vi "Main.vi"() -> ()   [LabVIEW 2015, in "Collect Data Mgr.lvlib"]
doc: "This template is based from the Queued Message Handler design pattern and the Queued Message Handler Project Template that ships with LabVIEW 2014.\n\nThe main difference is that the Queue is private to this module and communication between modules is done via Broadcast and Request events.\n\nRequest events are wrapped via public API methods and are handled in the Event handler loop in this VI.\nAny module can register for Broadcast events sent by this module.\n\nThe Event Handling Loop generates messages based on user interface actions.\n\nThe Message Handling Loop processes messages generated by the Event Handling Loop, or by other messages. The messages are string values, so new messages can be added easily to the Message Cases case structure in the Message Handling Loop. Each message cluster can also provide an optional value for Message Data, which is a variant that can be converted to whatever message-specific data is required.\n_____\nBased on Delacor QMH Project Template 2.1.0.2."
uses:
  Collect Data Mgr.lvlib
  <vilib>/Delacor/Delacor QMH/Libraries/Module Admin_class/Delacor_lib_QMH_Module Admin.lvclass
  Module Data--cluster.ctl
  <vilib>/Delacor/Delacor QMH/Libraries/Message Queue_class/Delacor_lib_QMH_Message Queue.lvclass/Delacor_lib_QMH_Message Queue.ctl
  Stop Argument--cluster.ctl
  <vilib>/Delacor/Delacor QMH/Libraries/Module Admin_class/Delacor_lib_QMH_Module Admin.lvclass/Delacor_lib_QMH_Module Admin.ctl
  Start Collect Argument--cluster.ctl
  Start Collect (Reply Payload)--cluster.ctl
  Stop Collect Argument--cluster.ctl
  Stop Collect (Reply Payload)--cluster.ctl
  Tool Interface/_HS Data Stream Params Cluster--typedef.ctl
  <vilib>/Delacor/Delacor QMH/Libraries/Message Queue_class/Delacor_lib_QMH_Enqueue Message (Single).vi
  <vilib>/Delacor/Delacor QMH/Libraries/Module Admin_class/Delacor_lib_QMH_Get External Launch.vi
  <vilib>/Utility/error.llb/Error Cluster From Error Code.vi
  <vilib>/ErrorRing/Error Ring.xnode
  <vilib>/Delacor/Delacor QMH/Libraries/Message Queue_class/Delacor_lib_QMH_Message Queue.lvclass
  Tool Interface/Tool Interface.lvlib
panel:
  in  "Stop":bool
  in  "Simulate MHL Error":bool
  in  "Simulate EHL Error":bool
  out "error out":errorcluster
  in  "Module Admin":refnum<class "Delacor_lib_QMH_Module Admin.lvclass">
  out "Status":string
  # "Other QMH Modules communicate with this Module via its Public API (wrappers for its Request Events).\n\nThis Module communicates with other Modules via its Broadcast Events.\nAny module that wants to get these messages, just registers for this module's Broadcast events."
  # "This template is for the Delacor Modified Queued Message Handler design pattern.\n\nSee the block diagram for more information on how to use this template."
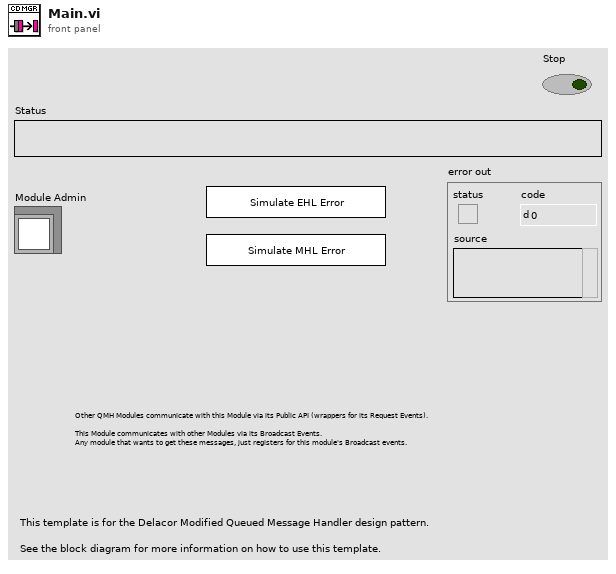
[diagram p1: front panel]
types:
  T1 = typedef "Collect Data Mgr.lvlib/Request Events--cluster.ctl" = cluster{"Stop Module":refnum<user-event>, "Show Panel":refnum<user-event>, "Hide Panel":refnum<user-event>, "Get Module Execution Status":refnum<user-event>, "Show Diagram":refnum<user-event>, "Start Collect":refnum<user-event>, "Stop Collect":refnum<user-event>}
  T2 = typedef "Collect Data Mgr.lvlib/Module Data--cluster.ctl" = cluster{"Status":string, "Error Code":u8, "Data Array DVR":refnum<data-value>, "Sample Data notifier":refnum<notifier>, "Block Count Notifier":refnum<notifier>, "Data Array":u32[][]}
  T3 = typedef "Collect Data Mgr.lvlib/Stop Argument--cluster.ctl" = cluster{"Origin":string, "Exit via Stop Module Req?":bool, "Wait for Module to stop?":bool}
  T4 = typedef "Collect Data Mgr.lvlib/Start Collect Argument--cluster.ctl" = cluster{"Lasers ON?":bool, "Move Length":i32, "Sample Data notifier":refnum<notifier>, "data value reference":refnum<data-value>, "Wait Notifier":refnum<notifier>}
  T5 = typedef "Collect Data Mgr.lvlib/Stop Collect Argument--cluster.ctl" = cluster{"dummy":bool, "Wait Notifier":refnum<notifier>}
  T6 = enum32{"Invalid", "Standard", "Closed", "Hidden", "Minimized", "Maximized"}
  T7 = enum16{"Idle", "Receive HS Data", "Close Connection"}
  T8 = typedef "Tool Interface.lvlib/_HS Data Stream Params Cluster--typedef.ctl" = cluster{"Raw Data Stream Loop cmd":enum16{"Idle", "Receive HS Data", "Close Connection"}, "Data Array DVR ref":refnum<data-value>, "Sample Data notifier":refnum<notifier>, "Block Count Notifier":refnum<notifier>}
  T9 = typedef "Collect Data Mgr.lvlib/Stop Collect (Reply Payload)--cluster.ctl" = cluster{"Success":bool, "CD_Status":i32, "Array Size":u32, "data value reference":refnum<data-value>}
  T10 = typedef "Tool Interface.lvlib/_Loop Ctrl Notifiers Cluster--typedef.ctl" = cluster{"Raw Stream Ctrl":refnum<notifier>}
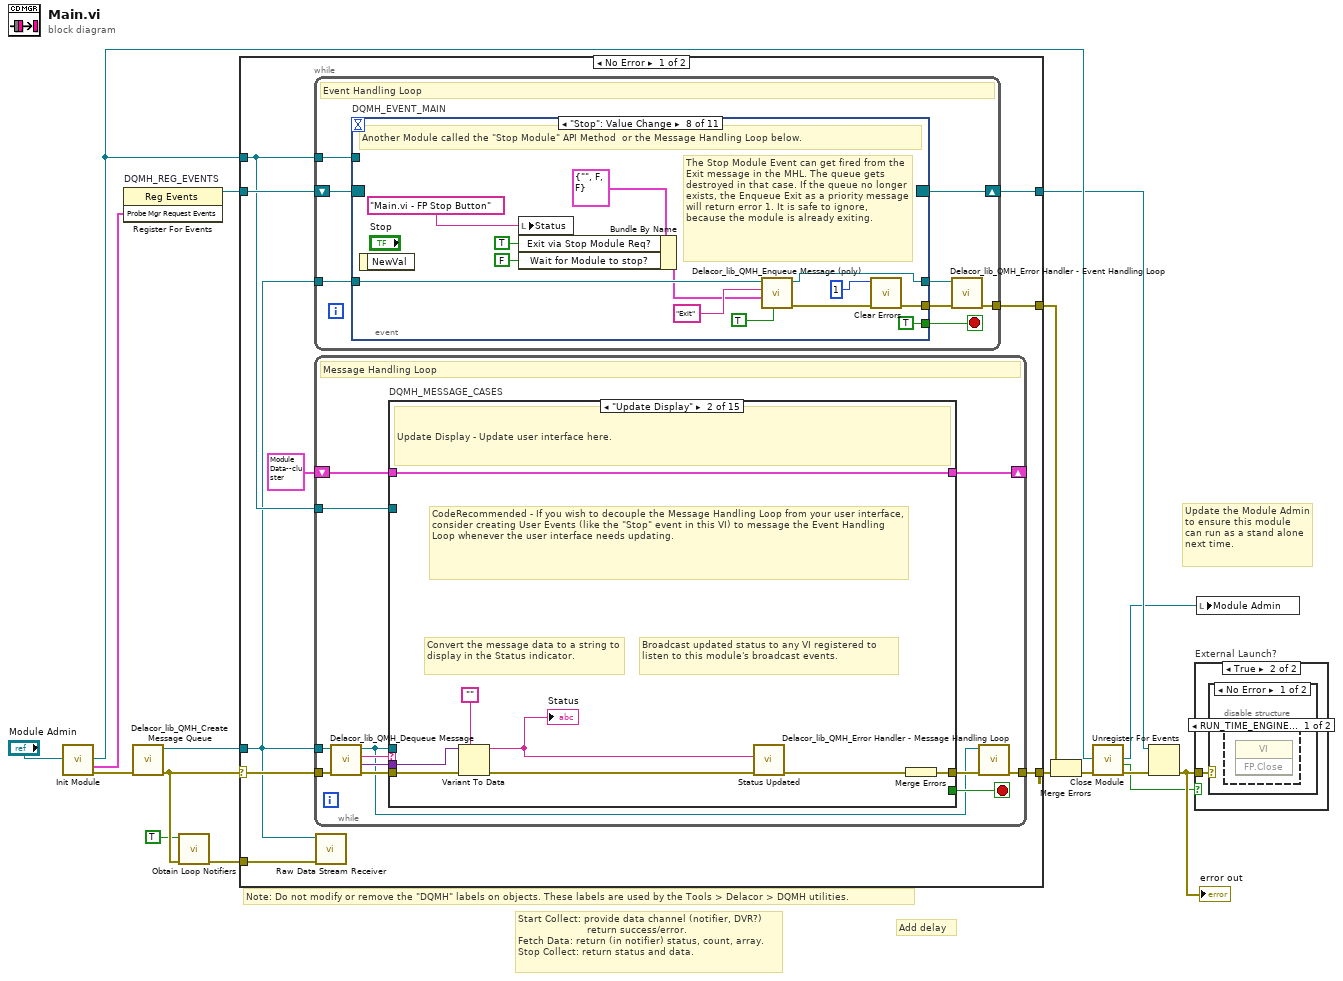
[diagram p0: block diagram]
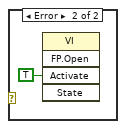
[diagram p4: hidden frame]
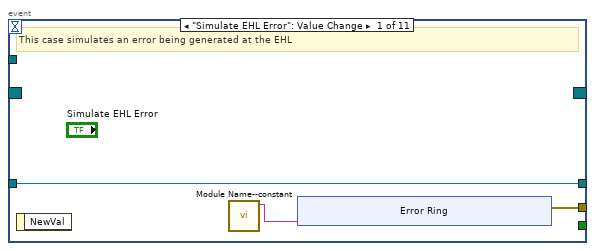
[diagram p5: hidden frame]
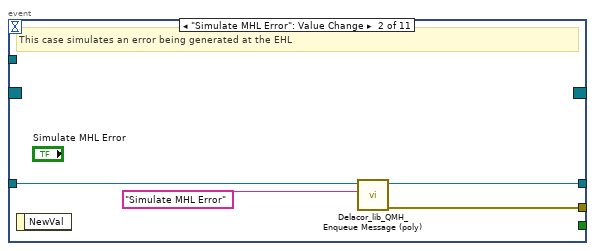
[diagram p6: hidden frame]
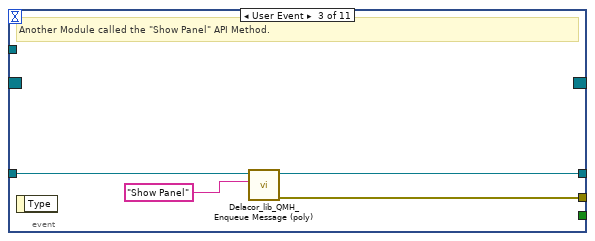
[diagram p7: hidden frame]
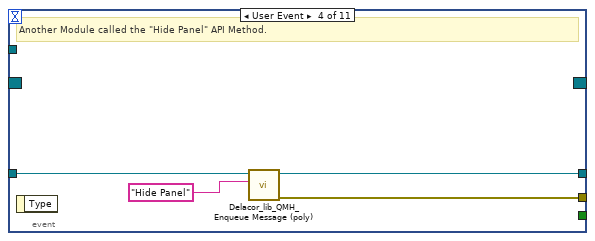
[diagram p8: hidden frame]
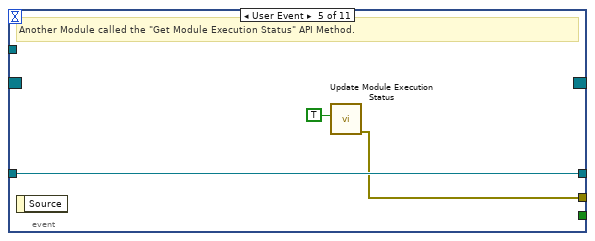
[diagram p9: hidden frame]
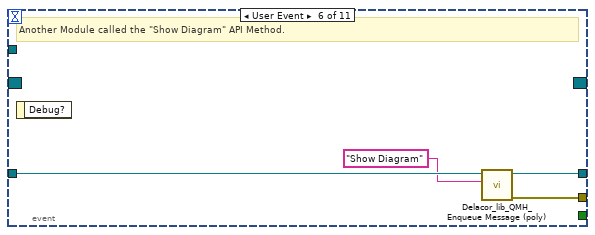
[diagram p10: hidden frame]
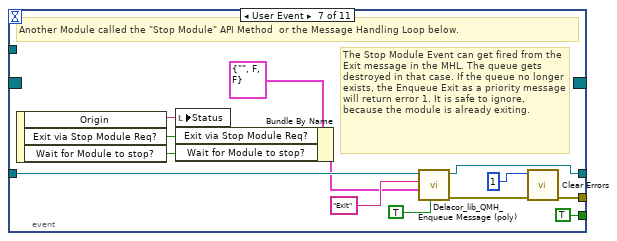
[diagram p11: hidden frame]
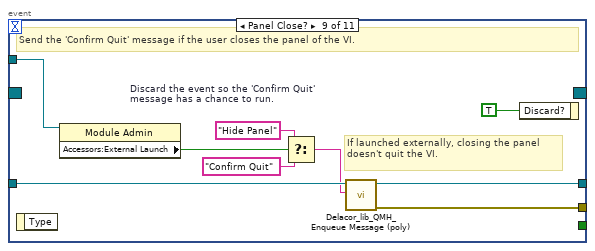
[diagram p12: hidden frame]
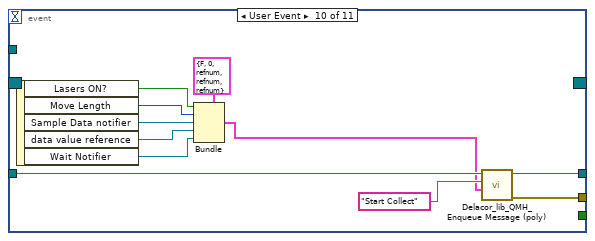
[diagram p13: hidden frame]
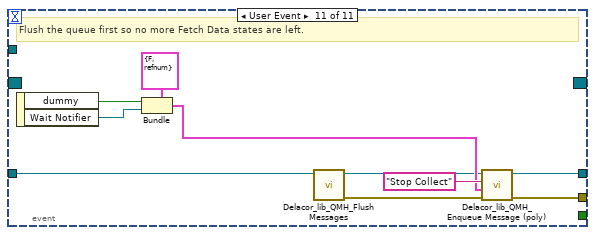
[diagram p14: hidden frame]
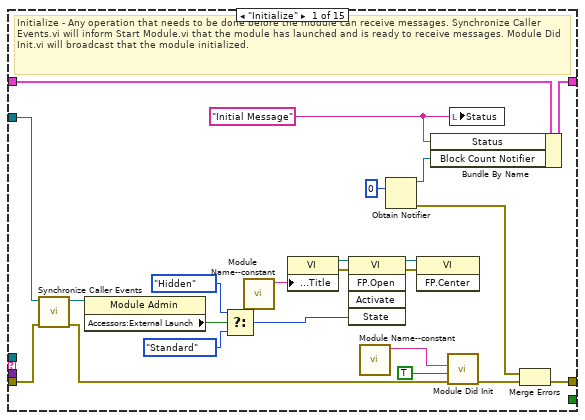
[diagram p15: hidden frame]
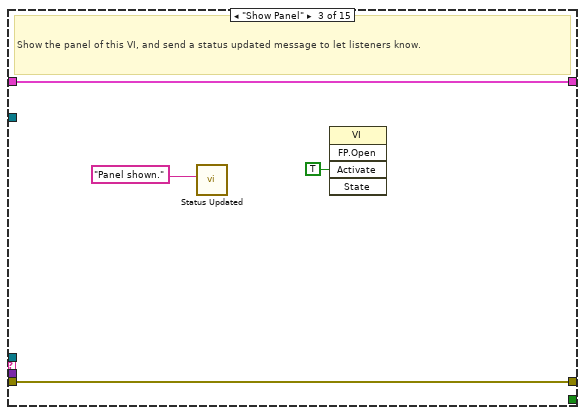
[diagram p16: hidden frame]
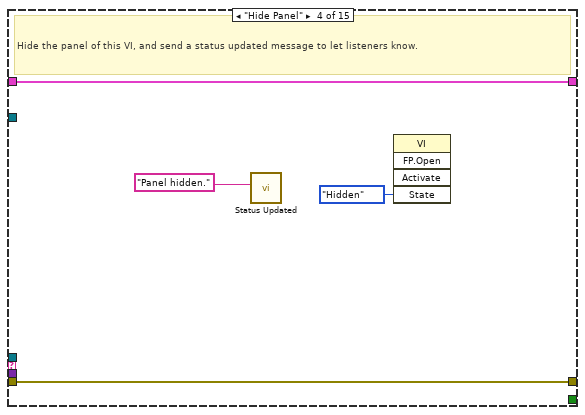
[diagram p17: hidden frame]
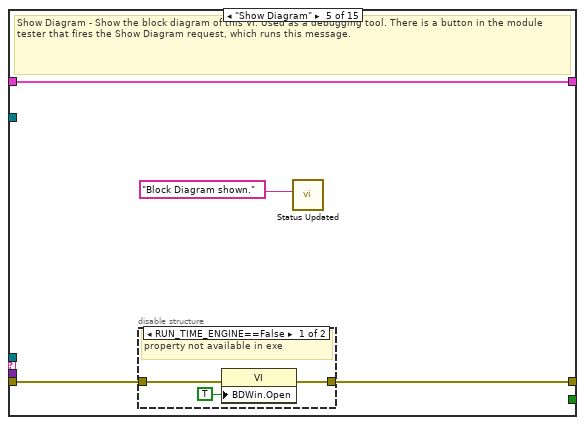
[diagram p18: hidden frame]
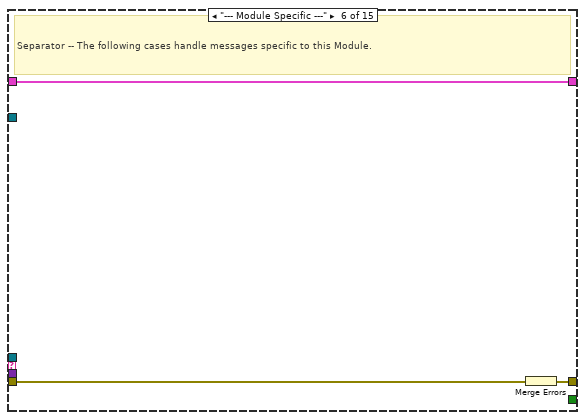
[diagram p20: hidden frame]
diagram:
  # "Add delay"
  # "Start Collect: provide data channel (notifier, DVR?)\n                       return success/error.\nFetch Data: return (in notifier) status, count, array.\nStop Collect: return status and data."
  # "Note: Do not modify or remove the \"DQMH\" labels on objects. These labels are used by the Tools > Delacor > DQMH utilities."
  # "Update the Module Admin to ensure this module can run as a stand alone next time."
  n1 = call "Init Module.vi"("Singleton Module Admin in"="Module Admin") -> ("error out"=w4:errorcluster, "Probe Mgr Request Events"=w13:T1, "Singleton Module Admin out"=w17:refnum<class "Delacor_lib_QMH_Module Admin.lvclass">)  [unwired: 8 in]
  n2 = register-events "DQMH_REG_EVENTS"(w13) -> (reference out=w14:refnum<event-registration>)  [unwired: 2 in, 1 out]
  n3 = call <vilib>:"Delacor_lib_QMH_Create Message Queue.vi"("error in (no error)"=w4) -> ("error out"=w3:errorcluster, "Message Queue"=w12:refnum<class "Delacor_lib_QMH_Message Queue.lvclass">)  [unwired: 9 in]
  n4 = call "Obtain Loop Notifiers.vi"("error in (no error)"=w3, "Create New"=TRUE) -> ("error out"=w1:errorcluster)  [unwired: 8 in, 1 out]
  n5 = case shown="No Error" w3 {
    selector: w3 -> [w21 w310]
    tunnel: [w26 w310] -> w16
    tunnel: [w25 w315] -> w15
    tunnel: w14 -> [w23 w315]
    tunnel: w12 -> [w18 _]
    tunnel: [w22 _] -> w8
    tunnel: w17 -> [w20 w311]
    tunnel: w1 -> [w19 _]
    frame No Error {
      n6 = while {
        tunnel: w18 -> [w34]
        shift-right: [w32] -> w25
        shift-left: w23 -> [w33]
        tunnel: [w28] -> w22
        tunnel: w20 -> [w27]
        stop <- w30 stop-if-true
        # "Event Handling Loop"
        n7 = event "DQMH_EVENT_MAIN" shown="[7] \"Stop\": Value Change" {
          selector: w33 -> [_ _ _ _ _ _ _ _ _ _ _]
          dyn-events: [_ _ _ _ _ _ _ _ _ _ _] -> w32
          timeout: _ -> [_ _ _ _ _ _ _ _ _ _ _]
          tunnel: [_ _ _ _ _ _ TRUE ("Discard?") TRUE ("Discard?") _ _ _] -> w30
          tunnel: w34 -> [w37 w48 w52 w56 w59 w63 w74 w87 w97 w109 w112]
          tunnel: [w36 w45 w50 w54 w58 w60 w68 w82 w96 w104 w115] -> w31
          tunnel: [w37 w47 w51 w55 w59 w62 w73 w86 w95 w108 w119] -> w29
          tunnel: w27 -> [_ _ _ _ _ _ _ _ w91 _ _]
          event "Simulate EHL Error": Value Change {
            # "This case simulates an error being generated at the EHL"
            n8 = event-data() -> ()  [unwired: 1 in, 1 out]
            n9 = call "Module Name--constant.vi"() -> ("Module Name"=w35:string)  [unwired: 11 in]
            n10 = xnode "Error Ring"("parameter 0"=w35) -> ("error out"=w36:errorcluster)
          }
          event "Simulate MHL Error": Value Change {
            # "This case simulates an error being generated at the EHL"
            n11 = event-data() -> ()  [unwired: 1 in, 1 out]
            n12 = call-poly <vilib>:"Delacor_lib_QMH_Enqueue Message (poly).vi"("Message"="Simulate MHL Error", "Message Queue in"=w48) -> ("error out"=w45:errorcluster, "Message Queue out"=w47:refnum<class "Delacor_lib_QMH_Message Queue.lvclass">)  [unwired: 8 in]
          }
          event User Event {
            # "Another Module called the \"Show Panel\" API Method."
            n13 = event-data() -> ()  [unwired: 1 in, 1 out]
            n14 = call-poly <vilib>:"Delacor_lib_QMH_Enqueue Message (poly).vi"("Message"="Show Panel", "Message Queue in"=w52) -> ("error out"=w50:errorcluster, "Message Queue out"=w51:refnum<class "Delacor_lib_QMH_Message Queue.lvclass">)  [unwired: 8 in]
          }
          event User Event {
            # "Another Module called the \"Hide Panel\" API Method."
            n15 = event-data() -> ()  [unwired: 1 in, 1 out]
            n16 = call-poly <vilib>:"Delacor_lib_QMH_Enqueue Message (poly).vi"("Message"="Hide Panel", "Message Queue in"=w56) -> ("error out"=w54:errorcluster, "Message Queue out"=w55:refnum<class "Delacor_lib_QMH_Message Queue.lvclass">)  [unwired: 8 in]
          }
          event User Event {
            # "Another Module called the \"Get Module Execution Status\" API Method."
            n17 = event-data() -> ()  [unwired: 1 in, 1 out]
            n18 = call "Update Module Execution Status.vi"("Running?"=TRUE) -> ("error out"=w58:errorcluster)  [unwired: 10 in]
          }
          event User Event {
            # "Another Module called the \"Show Diagram\" API Method."
            n19 = event-data() -> ()  [unwired: 1 in, 1 out]
            n20 = call-poly <vilib>:"Delacor_lib_QMH_Enqueue Message (poly).vi"("Message"="Show Diagram", "Message Queue in"=w63) -> ("error out"=w60:errorcluster, "Message Queue out"=w62:refnum<class "Delacor_lib_QMH_Message Queue.lvclass">)  [unwired: 8 in]
          }
          event User Event {
            # "The Stop Module Event can get fired from the Exit message in the MHL. The queue gets destroyed in that case. If the queue no longer exists, the Enqueue Exit as a priority message will return error 1. It is safe to ignore, because the module is already exiting."
            # "Another Module called the \"Stop Module\" API Method  or the Message Handling Loop below."
            n21 = event-data() -> ("Origin"=w72:string, "Exit via Stop Module Req?"=w66:bool, "Wait for Module to stop?"=w65:bool)  [unwired: 1 in]
            n22 = local write "Status"(w72) -> ()
            n23 = Bundle By Name(cluster=T3 {"Origin"="", "Exit via Stop Module Req?"=FALSE, "Wait for Module to stop?"=FALSE} ("Stop Argument"), "Exit via Stop Module Req?"=w66, "Wait for Module to stop?"=w65) -> (w64:T3)
            n24 = call-poly <vilib>:"Delacor_lib_QMH_Enqueue Message (poly).vi"("Priority Message? (F)"=TRUE, "Message Data"=w64, "Message"="Exit", "Message Queue in"=w74) -> ("error out"=w69:errorcluster, "Message Queue out"=w73:refnum<class "Delacor_lib_QMH_Message Queue.lvclass">)  [unwired: 6 in]
            n25 = call <vilib>:"Clear Errors.vi"("error in (no error)"=w69, "specific error code to clear (0: all)"=1) -> ("error out"=w68:errorcluster)  [unwired: 4 in, 1 out]
          }
          event "Stop": Value Change {
            # "The Stop Module Event can get fired from the Exit message in the MHL. The queue gets destroyed in that case. If the queue no longer exists, the Enqueue Exit as a priority message will return error 1. It is safe to ignore, because the module is already exiting."
            # "Another Module called the \"Stop Module\" API Method  or the Message Handling Loop below."
            n26 = event-data() -> ()  [unwired: 1 in, 1 out]
            n27 = local write "Status"("Main.vi - FP Stop Button") -> ()
            n28 = Bundle By Name(cluster=T3 {"Origin"="", "Exit via Stop Module Req?"=FALSE, "Wait for Module to stop?"=FALSE} ("Stop Argument"), "Exit via Stop Module Req?"=TRUE, "Wait for Module to stop?"=FALSE) -> (w80:T3)
            n29 = call-poly <vilib>:"Delacor_lib_QMH_Enqueue Message (poly).vi"("Priority Message? (F)"=TRUE, "Message Data"=w80, "Message"="Exit", "Message Queue in"=w87) -> ("error out"=w83:errorcluster, "Message Queue out"=w86:refnum<class "Delacor_lib_QMH_Message Queue.lvclass">)  [unwired: 6 in]
            n30 = call <vilib>:"Clear Errors.vi"("error in (no error)"=w83, "specific error code to clear (0: all)"=1) -> ("error out"=w82:errorcluster)  [unwired: 4 in, 1 out]
          }
          event Panel Close? {
            w98 = TRUE  # Discard the event so the 'Confirm Quit' message has a chance to run.
            # "If launched externally, closing the panel doesn't quit the VI."
            # "Send the 'Confirm Quit' message if the user closes the panel of the VI."
            n31 = event-data() -> ()  [unwired: 1 in, 1 out]
            n32 = property class="Module Admin"(reference=w91) -> ("Accessors:External Launch"=w90:bool)  [unwired: 1 in, 2 out]
            n33 = Select(t="Hide Panel" ("Message"), s=w90, f="Confirm Quit" ("Message")) -> (s? t:f=w92:string)
            n34 = call-poly <vilib>:"Delacor_lib_QMH_Enqueue Message (poly).vi"("Message"=w92, "Message Queue in"=w97) -> ("error out"=w96:errorcluster, "Message Queue out"=w95:refnum<class "Delacor_lib_QMH_Message Queue.lvclass">)  [unwired: 8 in]
            n35 = event-data("Discard?"=w98) -> ()  [unwired: 1 in, 1 out]
          }
          event User Event {
            n36 = event-data() -> ("Lasers ON?"=w103:bool, "Move Length"=w102:i32, "Sample Data notifier"=w101:refnum<notifier>, "data value reference"=w100:refnum<data-value>, "Wait Notifier"=w99:refnum<notifier>)  [unwired: 1 in]
            n37 = Bundle(cluster=T4 {"Lasers ON?"=FALSE, "Move Length"=0, "Sample Data notifier"=refnum, "data value reference"=refnum, "Wait Notifier"=refnum} ("Start Collect Argument"), "Lasers ON?"=w103, "Move Length"=w102, "Sample Data notifier"=w101, "data value reference"=w100, "Wait Notifier"=w99) -> (w105:T4)
            n38 = call-poly <vilib>:"Delacor_lib_QMH_Enqueue Message (poly).vi"("Message Data"=w105, "Message"="Start Collect", "Message Queue in"=w109) -> ("error out"=w104:errorcluster, "Message Queue out"=w108:refnum<class "Delacor_lib_QMH_Message Queue.lvclass">)  [unwired: 7 in]
          }
          event User Event {
            # "Flush the queue first so no more Fetch Data states are left."
            n39 = event-data() -> ("dummy"=w114:bool, "Wait Notifier"=w113:refnum<notifier>)  [unwired: 1 in]
            n40 = Bundle(cluster=T5 {"dummy"=FALSE, "Wait Notifier"=refnum} ("Stop Collect Argument"), "dummy"=w114, "Wait Notifier"=w113) -> (w116:T5)
            n41 = call-dynamic "Delacor_lib_QMH_Flush Messages.vi"("Message Queue in"=w112) -> ("error out"=w110:errorcluster, "Message Queue out"=w111:refnum<class "Delacor_lib_QMH_Message Queue.lvclass">)  [unwired: 7 in, 2 out]
            n42 = call-poly <vilib>:"Delacor_lib_QMH_Enqueue Message (poly).vi"("error in (no error)"=w110, "Message Data"=w116, "Message"="Stop Collect", "Message Queue in"=w111) -> ("error out"=w115:errorcluster, "Message Queue out"=w119:refnum<class "Delacor_lib_QMH_Message Queue.lvclass">)  [unwired: 6 in]
          }
        }
        n43 = call-dynamic "Delacor_lib_QMH_Error Handler - Event Handling Loop.vi"("error in (no error)"=w31, "Message Queue in"=w29) -> ("dup error in"=w28:errorcluster)  [unwired: 8 in, 1 out]
      }
      n44 = while {
        tunnel: w18 -> [w123]
        shift-right: [w129] -> _
        shift-left: T2 {"Status"="", "Error Code"=0, "Data Array DVR"=refnum, "Sample Data notifier"=refnum, "Block Count Notifier"=refnum, "Data Array"=[]} ("Data Cluster") -> [w130]
        tunnel: w21 -> [w127]
        tunnel: [w121] -> w26
        tunnel: w20 -> [w120]
        stop <- w128 stop-if-true
        # "Message Handling Loop"
        n45 = call-dynamic "Delacor_lib_QMH_Dequeue Message.vi"("error in (no error)"=w127, "Message Queue in"=w123) -> ("error out"=w126:errorcluster, "Message Data"=w124:variant, "Message"=w125:string, "Message Queue out"=w122:refnum<class "Delacor_lib_QMH_Message Queue.lvclass">)  [unwired: 6 in]
        n46 = case "DQMH_MESSAGE_CASES" shown="\"Update Display\"" w125 {
          selector: w125 -> [_ _ _ _ _ _ _ _ _ _ _ _ _ _ w297]
          tunnel: w122 -> [_ _ _ _ _ _ _ _ _ _ _ w255 w270 w293 _]
          tunnel: w126 -> [w144 w160 w166 w170 w173 w181 w201 _ w236 w239 w244 w261 w274 w295 _]
          tunnel: [w135 w161 w166 w170 w172 w179 w199 w232 w234 w237 w242 w252 w272 w290 w298] -> w131
          tunnel: w130 -> [w143 w162 w165 w169 w174 w180 w184 w217 w235 w238 w243 w260 w273 w277 w299]
          tunnel: [w142 w162 w165 w169 w174 w180 w183 w217 w235 w238 w243 w260 w273 w277 w299] -> w129
          tunnel: [_ _ _ _ _ _ _ _ _ _ _ _ _ w292 _] -> w128
          tunnel: w124 -> [_ w159 _ _ _ _ w200 w231 _ _ _ w259 _ w289 _]
          tunnel: w120 -> [w145 _ _ _ _ _ _ _ _ _ _ w254 _ w283 _]
          frame "Initialize" {
            w141 = "Initial Message" ("Initial Message")
            # "Initialize - Any operation that needs to be done before the module can receive messages. Synchronize Caller Events.vi will inform Start Module.vi that the module has launched and is ready to receive messages. Module Did Init.vi will broadcast that the module initialized."
            n47 = call "Synchronize Caller Events.vi"("error in (no error)"=w144, "Singleton Module Admin in"=w145) -> ("error out"=w138:errorcluster, "Singleton Module Admin out"=w136:refnum<class "Delacor_lib_QMH_Module Admin.lvclass">)  [unwired: 8 in]
            n48 = property class="Module Admin"(reference=w136) -> ("Accessors:External Launch"=w149:bool)  [unwired: 1 in, 2 out]
            n49 = Select(t=T6."Hidden" ("State"), s=w149, f=T6."Standard" ("State")) -> (s? t:f=w146:T6)
            n50 = call "Module Name--constant.vi"() -> ("Module Name"=w154:string)  [unwired: 11 in]
            n51 = property class="VI"("Front Panel.Title"=w154) -> (reference out=w152:refnum<vi>, error out=w153:errorcluster)  [unwired: 2 in]
            n52 = invoke class="VI" method="FP.Open"(reference=w152, error in=w153, "State"=w146) -> (reference out=w151:refnum<vi>, error out=w150:errorcluster)  [unwired: 2 in, 3 out]
            n53 = call "Module Name--constant.vi"() -> ("Module Name"=w139:string)  [unwired: 11 in]
            n54 = Obtain Notifier(notification data type=u32 0) -> (notifier out=w132:refnum<notifier>, error out=w134:errorcluster)  [unwired: 3 in, 1 out]
            n55 = invoke class="VI" method="FP.Center"(reference=w151, error in=w150) -> ()  [unwired: 1 in, 3 out]
            n56 = Bundle By Name(cluster=w143, "Status"=w141, "Block Count Notifier"=w132) -> (w142:T2)
            n57 = call "Module Did Init.vi"("error in (no error)"=w138, "Initialized?"=TRUE, "Origin"=w139) -> ("error out"=w137:errorcluster)  [unwired: 8 in]
            n58 = local write "Status"(w141) -> ()
            n59 = Merge Errors(w134, w137) -> (w135:errorcluster)
          }
          frame "Update Display" {
            # "Broadcast updated status to any VI registered to listen to this module's broadcast events."
            # "Convert the message data to a string to display in the Status indicator."
            # "CodeRecommended - If you wish to decouple the Message Handling Loop from your user interface, consider creating User Events (like the \"Stop\" event in this VI) to message the Event Handling Loop whenever the user interface needs updating."
            # "Update Display - Update user interface here."
            n60 = Variant To Data(error in=w160, type="", Variant=w159) -> (data=w157:string, error out=w156:errorcluster)
            "Status" <- w157
            n61 = call "Status Updated.vi"("error in (no error)"=w156, "Status"=w157) -> ("error out"=w155:errorcluster)  [unwired: 9 in]
            n62 = Merge Errors(w155) -> (w161:errorcluster)
          }
          frame "Show Panel" {
            # "Show the panel of this VI, and send a status updated message to let listeners know."
            n63 = call "Status Updated.vi"("Status"="Panel shown." ("format string")) -> ()  [unwired: 10 in, 1 out]
            n64 = invoke class="VI" method="FP.Open"("Activate"=TRUE ("Activate?")) -> ()  [unwired: 4 in, 5 out]
          }
          frame "Hide Panel" {
            # "Hide the panel of this VI, and send a status updated message to let listeners know."
            n65 = call "Status Updated.vi"("Status"="Panel hidden." ("format string")) -> ()  [unwired: 10 in, 1 out]
            n66 = invoke class="VI" method="FP.Open"("State"=T6."Hidden") -> ()  [unwired: 4 in, 5 out]
          }
          frame "Show Diagram" {
            # "Show Diagram - Show the block diagram of this VI. Used as a debugging tool. There is a button in the module tester that fires the Show Diagram request, which runs this message."
            n67 = disable-structure shown="RUN_TIME_ENGINE==False" {
              disable-tunnel: [w176 w178] -> w172
              disable-tunnel: w173 -> [w175 w178]
              frame condition #0 (active) {
                # "property not available in exe"
                n68 = property class="VI"(error in=w175, "BDWin.Open"=TRUE ("Block Diagram Window:Open")) -> (error out=w176:errorcluster)  [unwired: 1 in, 1 out]
              }
              frame condition #1 {
              }
            }
            n69 = call "Status Updated.vi"("Status"="Block Diagram shown." ("format string")) -> ()  [unwired: 10 in, 1 out]
          }
          frame "--- Module Specific ---" {
            # "Separator -- The following cases handle messages specific to this Module."
            n70 = Merge Errors(w181) -> (w179:errorcluster)
          }
          frame "Start Collect" {
            # "Set the Mode, move length, and the expected return data array length, and then start the data collection. Save the current VISA timeout value and set it to 1000mSec for data collection. Save the VISA resource name and the DVR ref that holds the full data storage array (passed in from caller)."
            n71 = Variant To Data(error in=w201, type=T4 {"Lasers ON?"=FALSE, "Move Length"=0, "Sample Data notifier"=refnum, "data value reference"=refnum, "Wait Notifier"=refnum} ("Start Collect Argument"), Variant=w200) -> (data=w189:T4, error out=w197:errorcluster)
            n72 = Unbundle By Name(w184) -> ("Block Count Notifier"=w202:refnum<notifier>)
            n73 = Unbundle By Name(w189) -> ("Sample Data notifier"=w192:refnum<notifier>, "data value reference"=w185:refnum<data-value>, "Lasers ON?"=w182:bool)
            n74 = Unbundle By Name(w189) -> ("Move Length"=w188:i32, "Wait Notifier"=w187:refnum<notifier>)
            n75 = call "Obtain Loop Notifiers.vi"() -> ("Loop Ctrl Notifiers Cluster"=w196:T10)  [unwired: 10 in, 1 out]
            n76 = Bundle By Name(cluster=T8 {"Raw Data Stream Loop cmd"=enum."Idle", "Data Array DVR ref"=refnum, "Sample Data notifier"=refnum, "Block Count Notifier"=refnum} ("Cluster"), "Block Count Notifier"=w202, "Sample Data notifier"=w192, "Data Array DVR ref"=w185, "Raw Data Stream Loop cmd"=T7."Receive HS Data" ("HS Data Stream SM enum")) -> (w193:T8)
            n77 = Unbundle By Name(w196) -> ("Raw Stream Ctrl"=w195:refnum<notifier>)
            n78 = Bundle By Name(cluster=w184, "Data Array DVR"=w185) -> (w183:T2)
            n79 = Send Notification(notification=w193, notifier=w195) -> (error out=w186:errorcluster)  [unwired: 1 in, 1 out]
            n80 = call "Setup Start Collect.vi"("error in (no error)"=w186, "Lasers ON?"=w182, "Wait Notifier"=w187, "Move Length"=w188) -> ("error out"=w190:errorcluster)  [unwired: 6 in, 1 out]
            n81 = Merge Errors(w190, w197) -> (w199:errorcluster)
          }
          frame "Stop Collect" {
            w213 = FALSE ("Laser 1")
            # "5/4/16 JX: explicitly turn off the Lasers for safety."
            # "Send the stop data collection command."
            n82 = call "Obtain Loop Notifiers.vi"() -> ("error out"=w207:errorcluster, "Loop Ctrl Notifiers Cluster"=w222:T10)  [unwired: 10 in]
            n83 = Unbundle By Name(w217) -> ("Block Count Notifier"=w212:refnum<notifier>, "Data Array DVR"=w210:refnum<data-value>)
            n84 = Variant To Data(type=T5 {"dummy"=FALSE, "Wait Notifier"=refnum} ("Stop Collect Argument"), Variant=w231) -> (data=w229:T5, error out=w227:errorcluster)  [unwired: 1 in]
            n85 = Unbundle By Name(w222) -> ("Raw Stream Ctrl"=w206:refnum<notifier>)
            n86 = Bundle By Name(cluster=T8 {"Raw Data Stream Loop cmd"=enum."Idle", "Data Array DVR ref"=refnum, "Sample Data notifier"=refnum, "Block Count Notifier"=refnum} ("Cluster"), "Raw Data Stream Loop cmd"=T7."Idle" ("HS Data Stream SM enum")) -> (w220:T8)
            n87 = Unbundle By Name(w229) -> ("Wait Notifier"=w228:refnum<notifier>)
            n88 = Send Notification(notification=w220, notifier=w206, error in (no error)=w207) -> (error out=w205:errorcluster)  [unwired: 1 out]
            n89 = call "Wait(ms).vi"("error in (no error)"=w205, "milliseconds"=u32 100) -> ("error out"=w204:errorcluster)  [unwired: 9 in]
            n90 = call "Collect Data Stop.vi"("error in (no error)"=w204) -> ("error out"=w203:errorcluster)  [unwired: 10 in]
            n91 = Unbundle By Name(w203) -> ("status"=w225:bool, "code"=w226:i32)
            n92 = call "Laser Control.vi"("error in (no error)"=w203, "Laser 2"=w213, "Laser 1"=w213) -> ("error out"=w233:errorcluster)  [unwired: 8 in]
            n93 = Not(x=w225) -> (.not. x?=w224:bool)
            n94 = Get Notifier Status(notifier=w212, error in (no error)=w233) -> (current notification=w211:u32, error out=w209:errorcluster)  [unwired: 3 out]
            n95 = Bundle By Name(cluster=T9 {"Success"=FALSE, "CD_Status"=0, "Array Size"=0, "data value reference"=refnum} ("Stop Collect (Reply Payload)"), "Array Size"=w211, "data value reference"=w210, "Success"=w224, "CD_Status"=w226) -> (w223:T9)
            n96 = call "Motion Stop.vi"("error in (no error)"=w209, "Decel?"=FALSE) -> ("error out"=w208:errorcluster)  [unwired: 9 in]
            n97 = Send Notification(notification=w223, notifier=w228, error in (no error)=w227) -> (error out=w216:errorcluster)  [unwired: 1 out]
            n98 = Merge Errors(w208, w216) -> (w232:errorcluster)
          }
          frame "---Copy This Frame---" {
            # "Duplicate this frame when creating new messages.  Change this comment in the duplicated frame to describe this message."
            n99 = Merge Errors(w236) -> (w234:errorcluster)
          }
          frame "--- Exit and Error Handling---" {
            # "Separator - The following cases handle errors and exit messages."
            n100 = Merge Errors(w239) -> (w237:errorcluster)
          }
          frame "Simulate MHL Error" {
            # "Simulate an error occurring at the MHL"
            n101 = call "Module Name--constant.vi"() -> ("Module Name"=w241:string)  [unwired: 11 in]
            n102 = xnode "Error Ring"("parameter 0"=w241) -> ("error out"=w240:errorcluster)
            n103 = Merge Errors(w244, w240) -> (w242:errorcluster)
          }
          frame "Error" {
            # "CodeRecommended - If you ever change the name of this \"Error\" message, you'll need to update the name in the Check Loop Error.vi as well."
            # "CodeRecommended - If the module is running in standalone mode (External Launch = FALSE), this code will pop up an error dialog and call the 'Exit' message if an error occurs. Add more fine-grained error handling here."
            # "Error - Check the error message data and respond accordingly. This message is sent by the \"Error Handler\" VIs at the end of each loop in this application."
            n104 = property class="Module Admin"(reference=w254) -> ("Accessors:External Launch"=w253:bool)  [unwired: 1 in, 2 out]
            n105 = Variant To Data(error in=w261, type=errorcluster {"status"=FALSE, "code"=0, "source"=""} ("error constant"), Variant=w259) -> (data=w262:errorcluster, error out=w257:errorcluster)
            n106 = call "Error Reported.vi"("Error"=w262) -> ()  [unwired: 10 in, 1 out]
            n107 = case shown="True" w253 {
              tunnel: [w267 _] -> w256
              tunnel: w255 -> [w266 _]
              tunnel: w262 -> [w263 _]
              frame False {
                # "If the module is running standalone, then pop up an error dialog and call the \"Exit\" message."
                n108 = call <vilib>:"Simple Error Handler.vi"("error in (no error)"=w263) -> ()  [unwired: 4 in, 5 out]
                n109 = call-poly <vilib>:"Delacor_lib_QMH_Enqueue Message (poly).vi"("Priority Message? (F)"=TRUE, "Message"="Exit", "Message Queue in"=w266) -> ("error out"=w267:errorcluster)  [unwired: 7 in, 1 out]
              }
              frame True {
                # "If the module was launched externally, calling the Error Reported broadcast VI is the only action performed by the \"Error\" message. The module's caller can then process the error appropriately."
              }
            }
            n110 = Merge Errors(w257, w256) -> (w252:errorcluster)
            n111 = local write "error out"(w252) -> ()
          }
          frame "Confirm Quit" {
            # "Confirm Quit - Message that can confirm whether or not the user wants to exit the application."
            n112 = call-poly <vilib>:"Delacor_lib_QMH_Enqueue Message (poly).vi"("Priority Message? (F)"=TRUE, "error in (no error)"=w274, "Message"="Exit", "Message Queue in"=w270) -> ("error out"=w271:errorcluster)  [unwired: 6 in, 1 out]
            n113 = Merge Errors(w271) -> (w272:errorcluster)
          }
          frame "Exit" {
            w287 = 91  # 91: not all Exit messages will have an argument
            w292 = TRUE  # Stop the VI
            # "Release the message queue reference"
            # "Exit - Exit the application."
            n114 = Variant To Data(error in=w295, type=T3 {"Origin"="", "Exit via Stop Module Req?"=FALSE, "Wait for Module to stop?"=FALSE} ("Stop Argument"), Variant=w289) -> (data=w285:T3, error out=w288:errorcluster)
            n115 = call <vilib>:"Clear Errors.vi"("error in (no error)"=w288, "specific error code to clear (0: all)"=w287) -> ("error out"=w294:errorcluster)  [unwired: 4 in, 1 out]
            n116 = Unbundle By Name(w277) -> ("Block Count Notifier"=w275:refnum<notifier>)
            n117 = call "Obtain Loop Notifiers.vi"() -> ("error out"=w280:errorcluster, "Loop Ctrl Notifiers Cluster"=w282:T10)  [unwired: 10 in]
            n118 = control-ref of="This VI"() -> (w284:refnum<vi>)
            n119 = Unbundle By Name(w282) -> ("Raw Stream Ctrl"=w281:refnum<notifier>)
            n120 = call-dynamic "Delacor_lib_QMH_Release Message Queue.vi"("error in (no error)"=w294, "Message Queue"=w293) -> ("error out"=w291:errorcluster)  [unwired: 9 in]
            n121 = call "Handle Exit.vi"("Stop Argument"=w285, "Admin in"=w283, "VI reference"=w284) -> ("error out"=w279:errorcluster)  [unwired: 7 in, 1 out]
            n122 = Release Notifier(notifier=w281, error in (no error)=w280) -> (error out=w278:errorcluster)  [unwired: 1 in, 2 out]
            n123 = Release Notifier(notifier=w275) -> (error out=w276:errorcluster)  [unwired: 2 in, 2 out]
            n124 = Merge Errors(w279, w276, w278, w291) -> (w290:errorcluster)
          }
          frame Default {
            # "'Default' case only runs if there is a message that isn't defined in any of the other cases.  Output a programming error."
            n125 = call "Module Name--constant.vi"() -> ("Module Name"=w296:string)  [unwired: 11 in]
            n126 = xnode "Error Ring"("parameter 0"=w297, "parameter 1"=w296) -> ("error out"=w298:errorcluster)
          }
        }
        n127 = call-dynamic "Delacor_lib_QMH_Error Handler - Message Handling Loop.vi"("error in (no error)"=w131, "Message Queue in"=w122) -> ("dup error in"=w121:errorcluster)  [unwired: 8 in, 1 out]
      }
      n128 = call "Raw Data Stream Receiver.vi"("error in (no error)"=w19, "Message Queue in"=w18) -> ()  [unwired: 10 in]
    }
    frame Error {
      # "Synchronize Caller Events.vi will inform Start Module.vi that the module has launched and will let the code calling Start Module.vi register for broadcasts and would permit the caller receive the broadcast that an error occurred at launch time."
      n129 = call "Synchronize Caller Events.vi"("Singleton Module Admin in"=w311) -> ("error out"=w308:errorcluster)  [unwired: 9 in, 1 out]
      n130 = call "Module Name--constant.vi"() -> ("Module Name"=w314:string)  [unwired: 11 in]
      n131 = Format Into String(format string="An error occurred during initialization. %s is no longer running.", w314) -> (resulting string=w312:string)  [unwired: 2 in, 1 out]
      n132 = Merge Errors(w310, w308) -> (w309:errorcluster)
      n133 = call "Error Reported.vi"("Additional Information"=w312, "Error"=w309) -> ()  [unwired: 9 in, 1 out]
    }
  }
  n134 = Merge Errors(w8, w16) -> (w7:errorcluster)
  n135 = call "Close Module.vi"("error in (no error)"=w7, "Module Admin in"=w17) -> ("error out"=w10:errorcluster, "External Launch"=w5:bool, "Module Admin out"=w9:refnum<class "Delacor_lib_QMH_Module Admin.lvclass">)  [unwired: 7 in]
  n136 = Unregister For Events(event registration refnum=w15, error in=w10) -> (error out=w6:errorcluster)
  "error out" <- w6
  n137 = case "External Launch?" shown="True" w5 {
    tunnel: w6 -> [_ w316]
    frame False {
    }
    frame True {
      n138 = case shown="No Error" w316 {
        frame No Error {
          n139 = disable-structure shown="RUN_TIME_ENGINE==True" {
            frame condition #0 {
              n140 = invoke class="VI" method="FP.Close"() -> ()  [unwired: 3 in, 3 out]
            }
            frame condition #1 (active) {
            }
          }
        }
        frame Error {
          n141 = invoke class="VI" method="FP.Open"("Activate"=TRUE ("Activate?")) -> ()  [unwired: 4 in, 5 out]
        }
      }
    }
  }
  n142 = local write "Module Admin"(w9) -> ()
